vi "ExecuteJobOnce.vi"(8 "error in (no error)":errorcluster, 10 "Job name wo extension":string, 11 "SM1000-control in":T1) -> (0 "error out":errorcluster, 3 "SM1000-control out":T1)   [LabVIEW 2013, in "EC1000-control.lvlib" / "SM1000-control.lvclass"]
doc: "Starts the execution of a job one time.\n\nThe host must have taken control of the EC1000 using the 'TakeHostControl' command, and must have previously loaded a job from local ('LoadFlashJob') or USB based (LoadUSBJob) Flash storage prior to issuing this command. Job execution will begin immediately without waiting unless it was constructed with a 'WaitForIO' instruction. The job can be stopped at any time by issuing an 'Abort' command.\n\nCommand: <\"ExecuteJobOnce\">,<job-name> or 207,<job-name>\nReturns: \"0\"s"
uses:
  SM1000-control.lvclass
  Object-reference.ctl
  SM1000-control.lvclass/SM1000-control.ctl
  Custom-errors.ctl
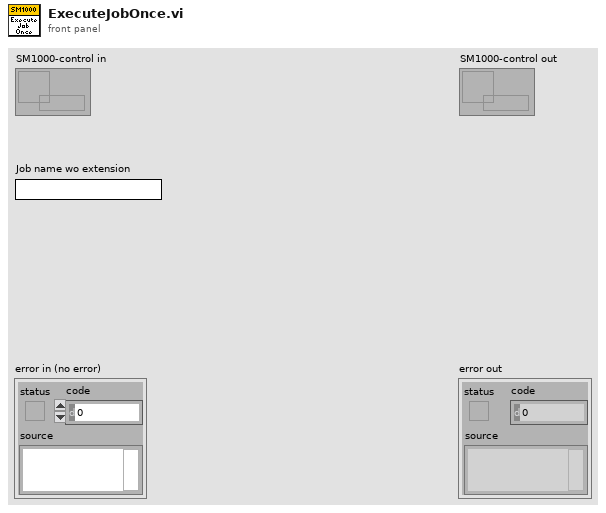
[diagram p1: front panel]
types:
  T1 = typedef "EC1000-control.lvlib/SM1000-control.lvclass/Object-reference.ctl" = refnum<data-value>
  T2 = typedef "EC1000-control.lvlib/SM1000-control.lvclass/Custom-errors.ctl" = enum16{"No error", "Not implemented", "Command not recognized", "Invalid input", "No connection", "Timeout", "Resource not loaded"}
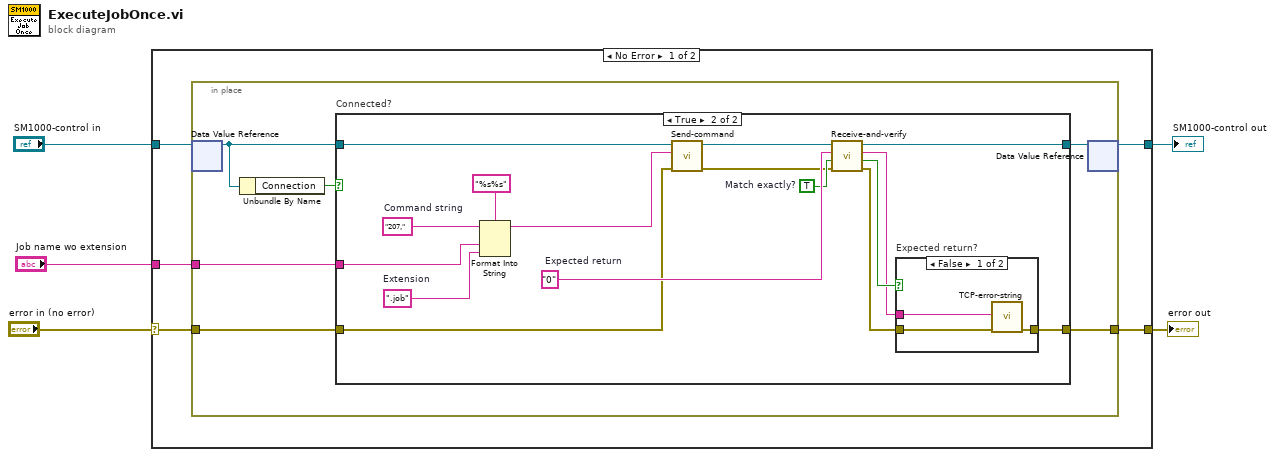
[diagram p0: block diagram]
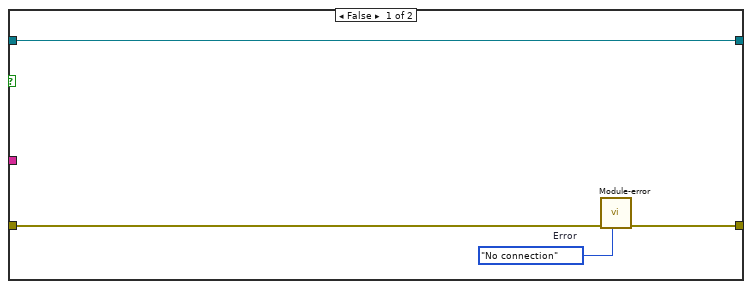
[diagram p2: hidden frame]
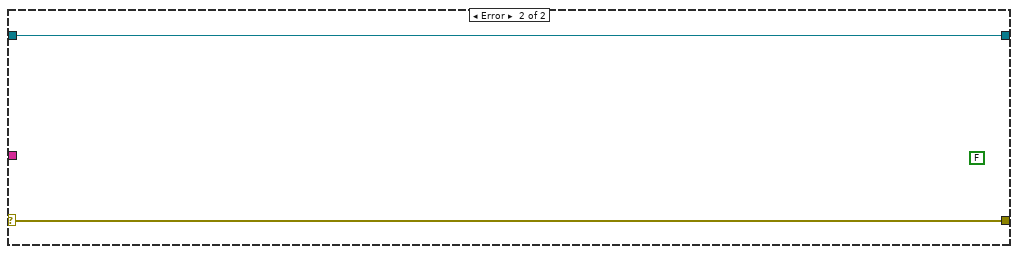
[diagram p4: hidden frame]
diagram:
  n1 = case shown="No Error" "error in (no error)" {
    selector: "error in (no error)" -> [w8 w42]
    tunnel: [w7 w42] -> w4
    tunnel: [w9 w41] -> w2
    tunnel: "SM1000-control in" -> [w10 w41]
    tunnel: "Job name wo extension" -> [w6 _]
    frame No Error {
      n2 = in-place {
        in-place-border: w8 -> [w16]
        in-place-border: [w13] -> w7
        in-place-border: w6 -> [w11]
        n3 = in-place-dvr #1(w10) -> (w14:refnum<class "SM1000-control.lvclass">)  [unwired: 1 out]
        n4 = Unbundle By Name(w14) -> ("Connection"=w15:bool)
        n5 = case "Connected?" shown="True" w15 {
          tunnel: w16 -> [w20 w29]
          tunnel: w14 -> [w18 w36]
          tunnel: [w19 w27] -> w13
          tunnel: [w18 w26] -> w12
          tunnel: w11 -> [_ w23]
          frame False {
            w17 = Custom-errors."No connection"  # Error
            n6 = call "Module-error.vi"("Error"=w17, "error in (no error)"=w20) -> ("error out"=w19:errorcluster)  [unwired: 9 in]
          }
          frame True {
            w22 = ".job"  # Extension
            w33 = TRUE  # Match exactly?
            w34 = "0"  # Expected return
            w25 = "207,"  # Command string
            n7 = Format Into String(format string="%s%s", initial string=w25, w23, w22) -> (resulting string=w24:string)  [unwired: 1 in, 1 out]
            n8 = call "Send-command.vi"("error in (no error)"=w29, "Command string"=w24, "SM1000-control in"=w36) -> ("error out"=w32:errorcluster, "SM1000-control out"=w35:refnum<class "SM1000-control.lvclass">)  [unwired: 7 in]
            n9 = call "Receive-and-verify.vi"("error in (no error)"=w32, "Match exactly?"=w33, "Expected return string"=w34, "SM1000-control in"=w35) -> ("error out"=w28:errorcluster, "Verified?"=w31:bool, "Return string"=w30:string, "SM1000-control out"=w26:refnum<class "SM1000-control.lvclass">)  [unwired: 4 in]
            n10 = case "Expected return?" shown="False" w31 {
              tunnel: w30 -> [w39 _]
              tunnel: w28 -> [w38 w40]
              tunnel: [w37 w40] -> w27
              frame False {
                n11 = call "TCP-error-string.vi"("error in (no error)"=w38, "Retun code"=w39) -> ("error out"=w37:errorcluster)  [unwired: 9 in]
              }
              frame True {
              }
            }
          }
        }
        n12 = in-place-dvr #1(w12) -> (w9:T1)  [unwired: 1 out]
      }
    }
    frame Error {
      (unwired) FALSE
    }
  }
  "error out" <- w4
  "SM1000-control out" <- w2
